vi "Quadrotor PC UDP Control.vi"() -> ()   [LabVIEW 2013]
uses:
  <vilib>/Utility/inputDevices.llb/closeJoystick.vi
  <vilib>/Utility/inputDevices.llb/joystickAcquire.vi
panel:
  out "Buffer OUT":u8[](array[numeric])=[204, 0, 0, 0, 0, 0, 0, 0, 0, 0, 0, 0, 0, 0, 0, 0, 0, 0, 0, 0, 0, 0, 0, 0, 0, 0, 0, 0, 0, 0, 0, 0, 85, 170] format="0x%x"
  out "axis info":T1 caption="坐标轴信息"
  in  "停止":bool
  out "油门":dbl(knob) scale=0.0..20000.0
  out "X axis":i32(slide) scale=-32768.0..32767.0
  out "Y axis":i32(slide) scale=32767.0..-32768.0
  in  "Buffer":u8[](array[numeric])=[204, 0, 0, 0, 0, 0, 0, 0, 0, 0, 0, 0, 0, 0, 0, 0, 0, 0, 0, 0, 0, 0, 0, 0, 0, 0, 0, 0, 0, 0, 0, 0, 85, 170] format="0x%x"
  out "XY图":cluster{i32[], i32[]}(graph)
  in  "启动控制":bool
  out "button info":T2 caption="按钮信息"
  out "direction info":T3 caption="方向信息"
  in  "ROLLoffset":i16
  in  "PITCHoffset":i16
  # "油门H"
  # "油门L"
  # "X轴H1"
  # "X轴H0"
  # "X轴L1"
  # "X轴L0"
  # "Y轴H1"
  # "Y轴H0"
  # "Y轴L1"
  # "Y轴L0"
  # "按钮9到12"
  # "按钮1到8"
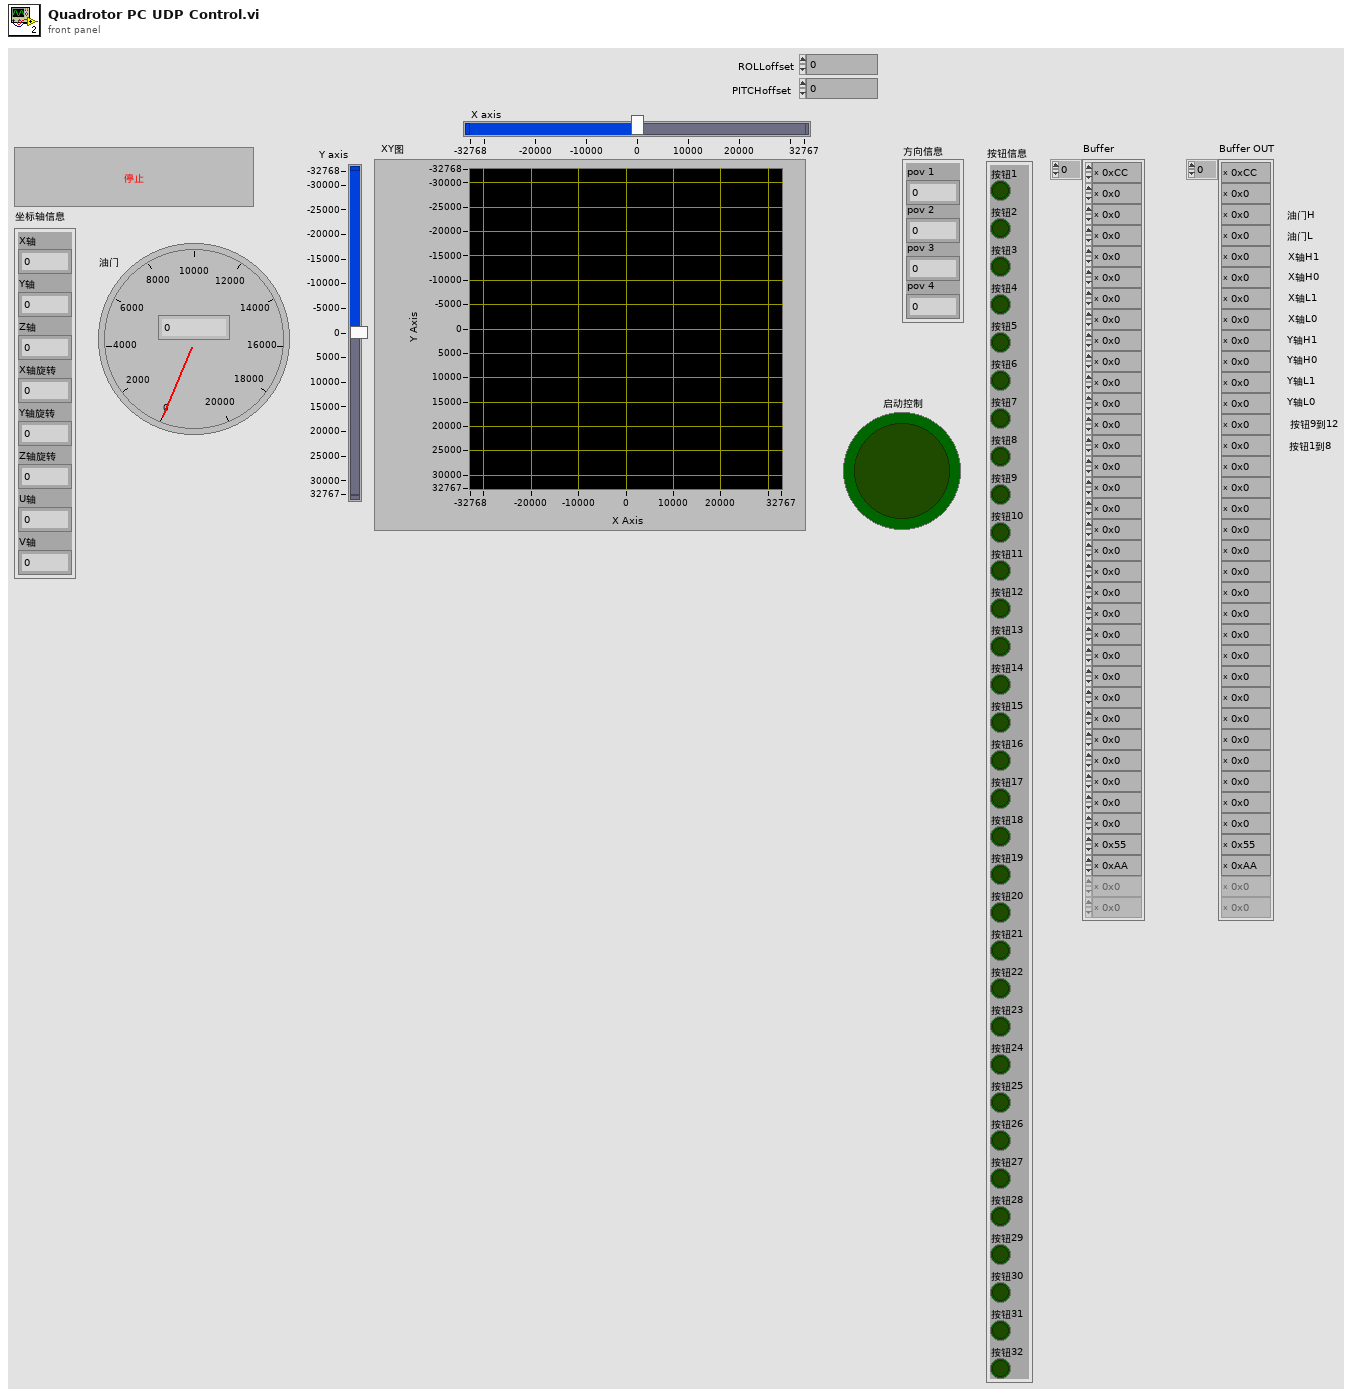
[diagram p1: front panel]
types:
  T1 = cluster{"X axis":i32, "Y axis":i32, "Z axis":i32, "X axis rotation":i32, "Y axis rotation":i32, "Z axis rotation":i32, "U axis":i32, "V axis":i32}
  T2 = cluster{"button 1":bool, "button 2":bool, "button 3":bool, "button 4":bool, "button 5":bool, "button 6":bool, "button 7":bool, "button 8":bool, "button 9":bool, "button 10":bool, "button 11":bool, "button 12":bool, "button 13":bool, "button 14":bool, "button 15":bool, "button 16":bool, "button 17":bool, "button 18":bool, "button 19":bool, "button 20":bool, "button 21":bool, "button 22":bool, "button 23":bool, "button 24":bool, "button 25":bool, "button 26":bool, "button 27":bool, "button 28":bool, "button 29":bool, "button 30":bool, "button 31":bool, "button 32":bool}
  T3 = cluster{"pov 1":i32, "pov 2":i32, "pov 3":i32, "pov 4":i32}
  T4 = cluster{"axes total":u32, "buttons total":u32, "pov total":u32, "device name":string}[]
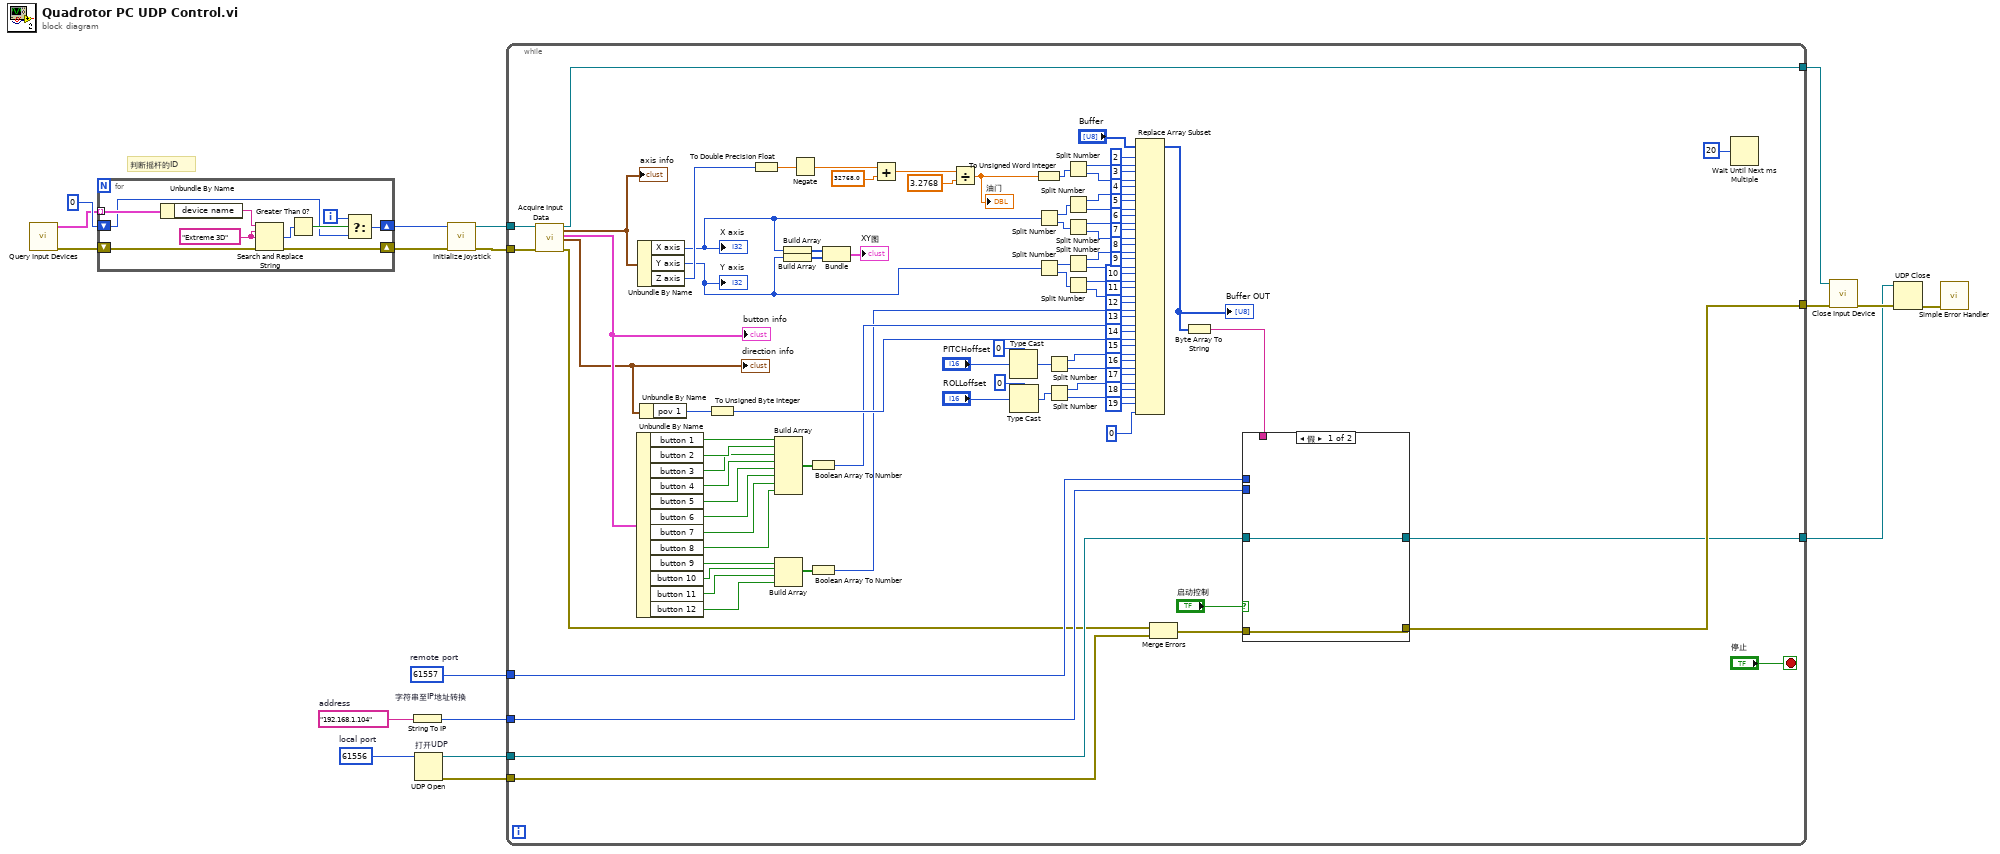
[diagram p0: block diagram]
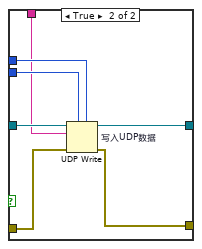
[diagram p2: hidden frame]
diagram:
  w7 = u16 61557  # remote port
  w8 = u16 61556  # local port
  w9 = "192.168.1.104"  # address
  # "判断摇杆的ID"
  n1 = call <vilib>:"Query Input Devices.vi"() -> ("error out"=w12:errorcluster, "joystick info"=w10:T4)  [unwired: 8 in, 2 out]
  n2 = for {
    tunnel: w10 -> [w28] mode=indexing
    shift-right: [w21] -> w13
    shift-left: 0 ("device index") -> [w22]
    shift-right: [w19] -> w11
    shift-left: w12 -> [w20]
    i -> [w23]
    w26 = "Extreme 3D" ("搜索字符串")
    n3 = Unbundle By Name(w28) -> ("device name"=w27:string)
    n4 = Search and Replace String ("搜索替换字符串")(input string=w27, search string=w26, replace string=w26, error in=w20) -> (number of replacements=w25:i32, error out=w19:errorcluster)  [unwired: 4 in, 2 out]
    n5 = Greater Than 0?(x=w25) -> (x > 0?=w24:bool)
    n6 = Select(t=w23, s=w24, f=w22) -> (s? t:f=w21:i32)
  }
  n7 = String To IP "字符串至IP地址转换"(1:w9) -> (0:w6:u32)
  n8 = UDP Open "打开UDP"(11:w8) -> (port=w5:refnum<k16>, 0:w4:errorcluster)  [unwired: 4 in, 1 out]
  n9 = call <vilib>:"Initialize Joystick.vi"("error in (no error)"=w11, "device index"=w13) -> ("error out"=w16:errorcluster, "device ID"=w18:refnum<k1>)  [unwired: 8 in]
  n10 = while {
    tunnel: w18 -> [w122]
    tunnel: [w121] -> w17
    tunnel: w16 -> [w113]
    tunnel: [w60] -> w15
    tunnel: w7 -> [w36]
    tunnel: w6 -> [w35]
    tunnel: w5 -> [w34]
    tunnel: w4 -> [w32]
    tunnel: [w29] -> w1
    stop <- "停止" stop-if-true
    n11 = call-poly <vilib>:"Acquire Input Data.vi"("device ID"=w122, "error in (no error)"=w113) -> ("device ID"=w121:refnum<k1>, "axis info"=w119:T1, "button info"=w82:T2, "direction info"=w65:T3, "error out"=w33:errorcluster)  [unwired: 13 in]
    "axis info" <- w119
    "button info" <- w82
    "direction info" <- w65
    n12 = Unbundle By Name(w82) -> ("button 1"=w79:bool, "button 2"=w78:bool, "button 3"=w77:bool, "button 4"=w76:bool, "button 5"=w75:bool, "button 6"=w74:bool, "button 7"=w73:bool, "button 8"=w72:bool, "button 9"=w70:bool, "button 10"=w69:bool, "button 11"=w68:bool, "button 12"=w67:bool)
    n13 = Unbundle By Name(w119) -> ("X axis"=w84:i32, "Y axis"=w89:i32, "Z axis"=w107:i32)
    "X axis" <- w84
    "Y axis" <- w89
    n14 = Unbundle By Name(w65) -> ("pov 1"=w64:i32)
    n15 = To Unsigned Byte Integer(number=w64) -> (unsigned 8bit integer=w61:u8)
    n16 = To Double Precision Float(number=w107) -> (double precision float=w114:dbl)
    n17 = Build Array(w79, w78, w77, w76, w75, w74, w73, w72) -> (w71:bool[])
    n18 = Build Array(w70, w69, w68, w67) -> (w66:bool[])
    n19 = Build Array(w84) -> (w109:i32[])
    n20 = Build Array(w89) -> (w108:i32[])
    n21 = Negate(x=w114) -> (-x=w115:dbl)
    n22 = Boolean Array To Number ("布尔数组至数值转换")(Boolean array=w71) -> (number=w43:u8)
    n23 = Boolean Array To Number ("布尔数组至数值转换")(Boolean array=w66) -> (number=w42:u8)
    n24 = Bundle(w109, w108) -> (→"XY图":cluster{i32[], i32[]})  [unwired: 1 in]
    n25 = Add(x=w115, y=32768.0) -> (x+y=w118:dbl)
    n26 = Divide(x=w118, y=3.2768) -> (x/y=w106:dbl)
    "油门" <- w106
    n27 = Type Cast(type=u16 0, x="PITCHoffset") -> (*(type *) &x=w50:u16)
    n28 = Type Cast(type=u16 0, x="ROLLoffset") -> (*(type *) &x=w47:u16)
    n29 = To Unsigned Word Integer(number=w106) -> (unsigned 16bit integer=w111:u16)
    n30 = Split Number(x=w84) -> (hi(x)=w101:u16, lo(x)=w100:u16)
    n31 = Split Number(x=w89) -> (hi(x)=w90:u16, lo(x)=w91:u16)
    n32 = Split Number(x=w50) -> (hi(x)=w49:u8, lo(x)=w48:u8)
    n33 = Split Number(x=w47) -> (hi(x)=w46:u8, lo(x)=w45:u8)
    n34 = Split Number(x=w111) -> (hi(x)=w41:u8, lo(x)=w40:u8)
    n35 = Split Number(x=w101) -> (hi(x)=w39:u8, lo(x)=w38:u8)
    n36 = Split Number(x=w100) -> (hi(x)=w99:u8, lo(x)=w98:u8)
    n37 = Split Number(x=w90) -> (hi(x)=w88:u8, lo(x)=w87:u8)
    n38 = Split Number(x=w91) -> (hi(x)=w86:u8, lo(x)=w85:u8)
    n39 = Replace Array Subset(array="Buffer", new element #1=w41, index #1=2 ("索引"), new element #2=w40, index #2=3 ("索引"), new element #3=w39, index #3=4 ("索引"), new element #4=w38, index #4=5 ("索引"), new element #5=w99, index #5=6 ("索引"), new element #6=w98, index #6=7 ("索引"), new element #7=w88, index #7=8 ("索引"), new element #8=w87, index #8=9 ("索引"), new element #9=w86, index #9=10 ("索引"), new element #10=w85, index #10=11 ("索引"), new element #11=w42, index #11=12 ("索引"), new element #12=w43, index #12=13 ("索引"), new element #13=w61, index #13=14 ("索引"), new element #14=w49, index #14=15 ("索引"), new element #15=w48, index #15=16 ("索引"), new element #16=w46, index #16=17 ("索引"), new element #17=w45, index #17=18 ("索引"), new element #18=u8 0 ("新元素/子数组"), index #18=19 ("索引")) -> (w37:u8[])
    "Buffer OUT" <- w37
    n40 = Merge Errors(w33, w32) -> (w31:errorcluster)
    n41 = Byte Array To String(unsigned byte array=w37) -> (string=w30:string)
    n42 = case shown="假" "启动控制" {
      tunnel: [w124 w127] -> w60
      tunnel: w36 -> [_ w131]
      tunnel: w35 -> [_ w130]
      tunnel: w34 -> [w123 w129]
      tunnel: w31 -> [w124 w128]
      tunnel: w30 -> [_ w126]
      tunnel: [w123 w125] -> w29
      frame False {
      }
      frame True {
        n43 = UDP Write "写入UDP数据"(address=w130, port or service name=w131, connection ID=w129, data in=w126, 8:w128) -> (error out=w127:errorcluster, 3:w125:refnum<k16>)  [unwired: 1 in]
      }
    }
    n44 = Wait Until Next ms Multiple(millisecond multiple=u32 20 ("毫秒倍数")) -> ()  [unwired: 1 out]
  }
  n45 = call-poly <vilib>:"Close Input Device.vi"("error in (no error)"=w15, "device ID"=w17) -> ("error out"=w2:errorcluster)  [unwired: 8 in]
  n46 = UDP Close(connection ID=w1, 8:w2) -> (error out=w3:errorcluster)  [unwired: 1 out]
  n47 = call <vilib>:"Simple Error Handler.vi"("error in (no error)"=w3) -> ()  [unwired: 4 in, 5 out]
